vi "Tn derivative recursive.vi"(1 "p-the derivative":i32, 2 "n":i32) -> (0 "Tn^p (0) array":i32[][](array[numeric]))   [LabVIEW 2020]
panel:
  # "Derivatives of Tn(x=0). When used for Chebyshev approximation,  f(x) contains another constant term."
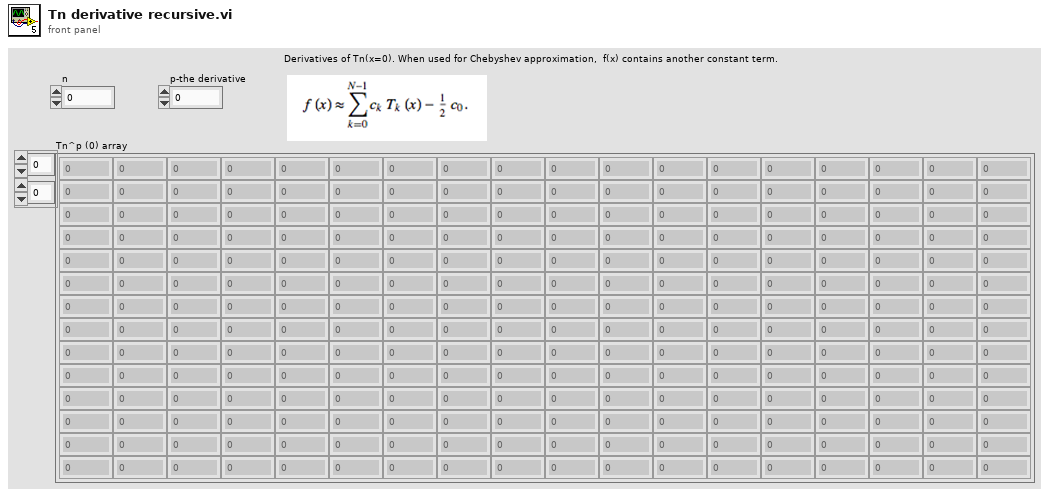
[diagram p1: front panel]
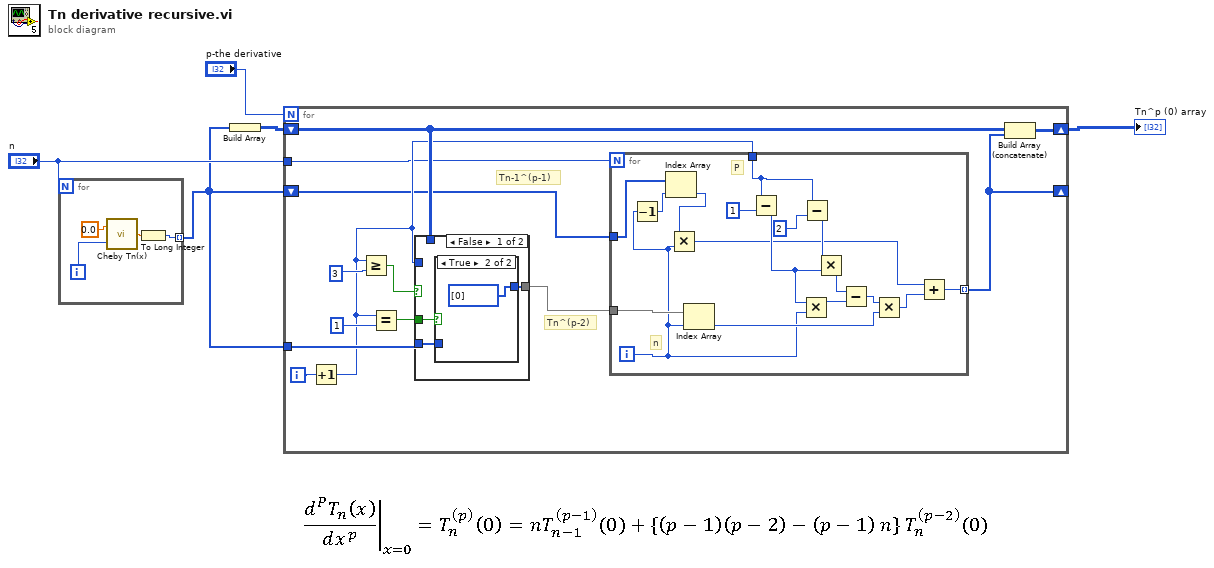
[diagram p0: block diagram]
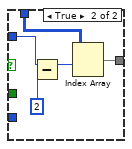
[diagram p3: hidden frame]
diagram:
  n1 = for {
    N: "n" -> [_]
    tunnel: [w6] -> w2 mode=indexing
    i -> [w9]
    n2 = call "Cheby Tn(x).vi"("n"=w9, "x"=0.0) -> ("T(n,x)"=w7:dbl)
    n3 = To Long Integer(number=w7) -> (32bit integer=w6:i32)
  }
  n4 = Build Array(w2) -> (w1:i32[][])
  n5 = for {
    N: "p-the derivative" -> [_]
    shift-right: [w10] -> _
    shift-left: w2 -> [w12]
    tunnel: "n" -> [w11]
    shift-right: [w22] -> w4
    shift-left: w1 -> [w20]
    tunnel: w2 -> [w15]
    i -> [w19]
    # "Tn^(p-2)"
    # "Tn-1^(p-1)"
    n6 = Increment(x=w19) -> (x+1=w14:i32)
    n7 = Greater Or Equal?(x=w14, y=3) -> (x >= y?=w21:bool)
    n8 = Equal?(x=w14, y=1) -> (x = y?=w16:bool)
    n9 = case shown="False" w21 {
      tunnel: w14 -> [_ w47]
      tunnel: w20 -> [_ w46]
      tunnel: [w42 w45] -> w13
      tunnel: w16 -> [w41 _]
      tunnel: w15 -> [w40 _]
      frame False {
        n10 = case shown="True" w41 {
          tunnel: [w43 i32[] [0]] -> w42
          tunnel: w40 -> [w43 _]
          frame False {
          }
          frame True {
          }
        }
      }
      frame True {
        n11 = Subtract(x=w47, y=2) -> (x-y=w49:i32)
        n12 = Index Array(array=w46, index (row)=w49) -> (element=w45:i32[])  [unwired: 1 in]
      }
    }
    n13 = for {
      N: w11 -> [_]
      tunnel: w12 -> [w39]
      tunnel: w13 -> [w36]
      tunnel: [w25] -> w10 mode=indexing
      tunnel: w14 -> [w24]
      i -> [w23]
      # "n"
      # "P"
      n14 = Decrement(x=w23) -> (x-1=w37:i32)
      n15 = Index Array(array=w39, index=w37) -> (element=w38:i32)
      n16 = Multiply(x=w38, y=w23) -> (x*y=w26:i32)
      n17 = Index Array(array=w36, index=w23) -> (element=w28:i32)
      n18 = Subtract(x=w24, y=u8 1) -> (x-y=w30:i32)
      n19 = Multiply(x=w30, y=w23) -> (x*y=w31:i32)
      n20 = Subtract(x=w24, y=u8 2) -> (x-y=w33:i32)
      n21 = Multiply(x=w33, y=w30) -> (x*y=w32:i32)
      n22 = Subtract(x=w32, y=w31) -> (x-y=w29:i32)
      n23 = Multiply(x=w29, y=w28) -> (x*y=w27:i32)
      n24 = Add(x=w26, y=w27) -> (x+y=w25:i32)
    }
    n25 = Build Array (concatenate)(w20, w10) -> (w22:i32[][])
  }
  "Tn^p (0) array" <- w4
